vi "Untitled 9.vi"(8 "error in (no error)":errorcluster, 11 "AddStringGcodeToList in":refnum<class "XuLyDataDisplay.lvclass">) -> (0 "error out":errorcluster, 3 "AddStringGcodeToList out":refnum<class "XuLyDataDisplay.lvclass">)   [LabVIEW 2017]
uses:
  ClassParameter/ParameterConf.lvclass
  stateLoopEvent.ctl
  XuLyDataDisplay.lvclass
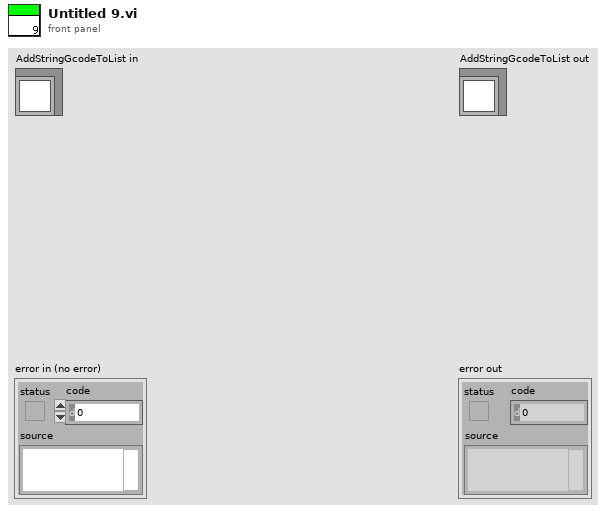
[diagram p1: front panel]
types:
  T1 = typedef "stateLoopEvent.ctl" = enum16{"Running", "init", "End"}
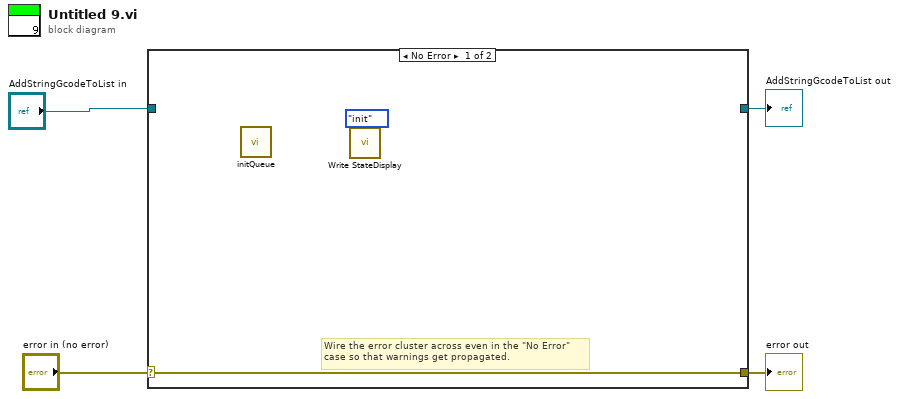
[diagram p0: block diagram]
diagram:
  n1 = case shown="No Error" "error in (no error)" {
    selector: "error in (no error)" -> [w6 w8]
    tunnel: [w6 w8] -> w3
    tunnel: [_ w7] -> w1
    tunnel: "AddStringGcodeToList in" -> [_ w7]
    frame No Error {
      # "Wire the error cluster across even in the \"No Error\"\ncase so that warnings get propagated."
      n2 = call-dynamic "initQueue.vi"() -> ()  [unwired: 10 in, 2 out]
      n3 = call-dynamic "Write StateDisplay.vi"("stateLoopEvent"=stateLoopEvent."init") -> ()  [unwired: 9 in, 2 out]
    }
    frame Error {
    }
  }
  "error out" <- w3
  "AddStringGcodeToList out" <- w1
